vi "Tracking_voltmeter.vi"() -> ()   [LabVIEW 2021]
uses:
  Main states enum-tracking.ctl
  Globals/Global message.vi
  Globals/CH1.vi
  Globals/CH2.vi
  Globals/CH3.vi
  Globals/CH4.vi
  Globals/CH5.vi
panel:
  in  "Time base [ms]":u32=100
  out "DOWN":bool
  out "UP":bool
  in  "ADC resolution":i32=5
  in  "ADC ref":dbl=5.0
  in  "Input channel":enum16{"CH1", "CH2", "CH3", "CH4", "CH5"}(ring)
  out "Waveform Chart":dynamicdata(graph)=[{"t0"=timestamp(3758015842.540576 s since 1904-01-01), "dt"=1.0, "Y"=[1.9925690374558243]}, {"t0"=timestamp(3758015842.540576 s since 1904-01-01), "dt"=1.0, "Y"=[2.03125]}]
  out "Uo ADC":dbl format="%_3g"
  out "Brojac":i32
  out "Indicator":dbl format="%_3g"
  in  "Stop Button":bool
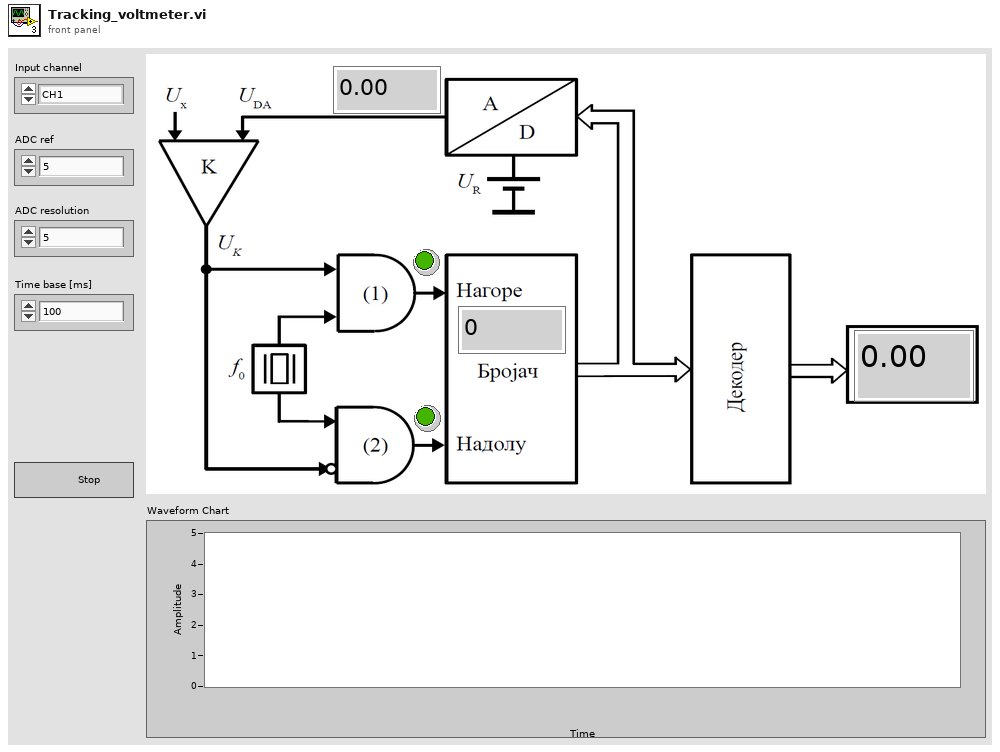
[diagram p1: front panel]
types:
  T1 = typedef "Main states enum-tracking.ctl" = enum16{"Initialize", "Update", "Stop"}
  T2 = cluster{"Voltage":dbl, "Current":dbl, "Message":string}
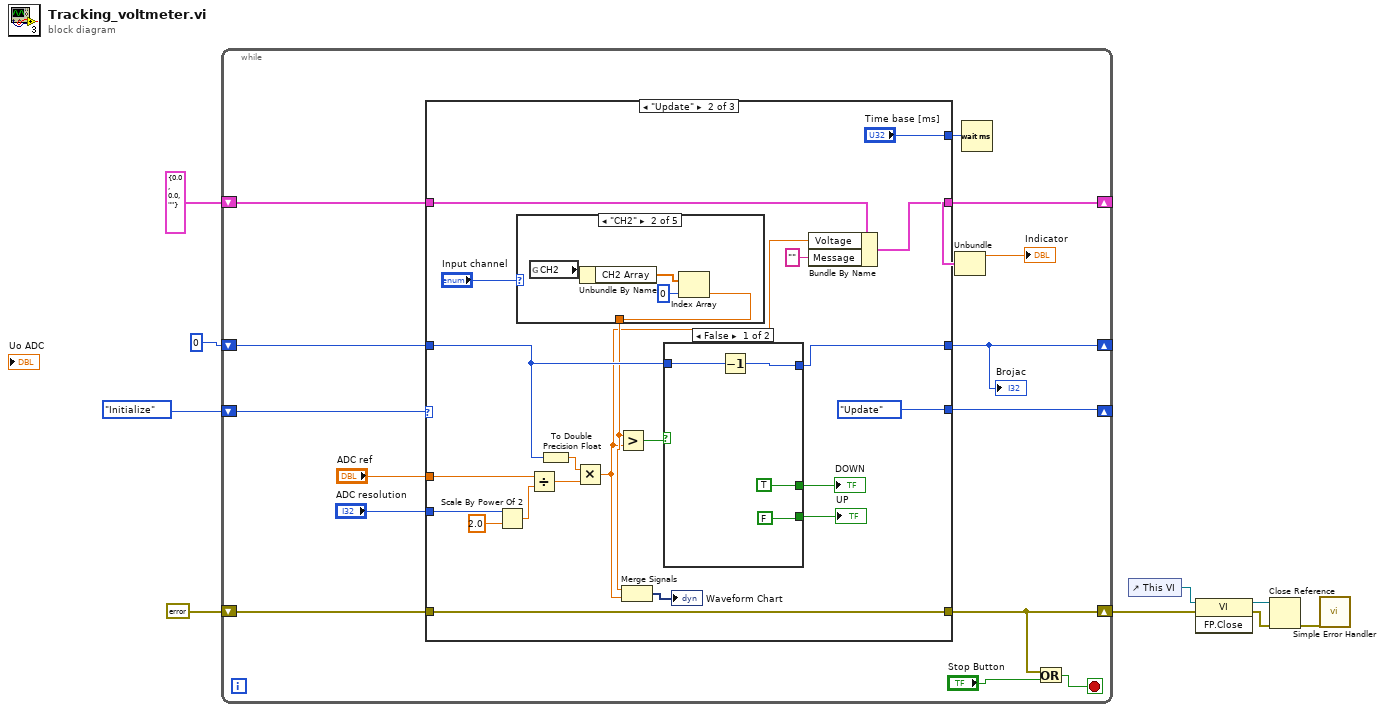
[diagram p0: block diagram]
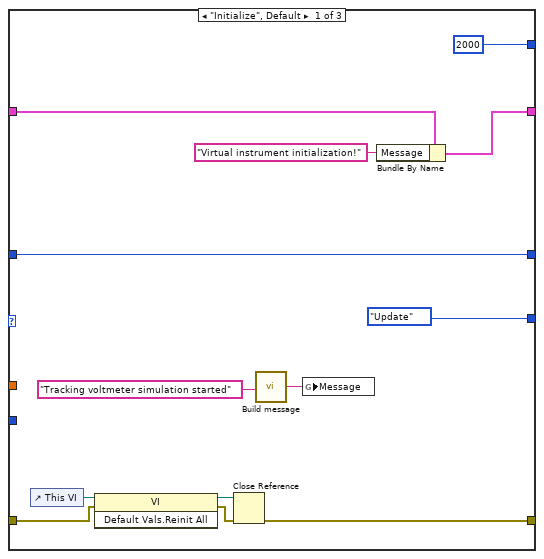
[diagram p2: hidden frame]
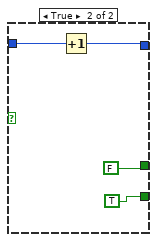
[diagram p3: hidden frame]
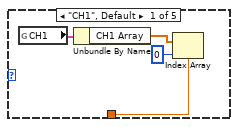
[diagram p4: hidden frame]
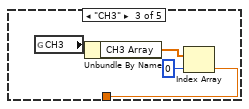
[diagram p5: hidden frame]
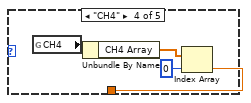
[diagram p6: hidden frame]
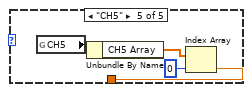
[diagram p7: hidden frame]
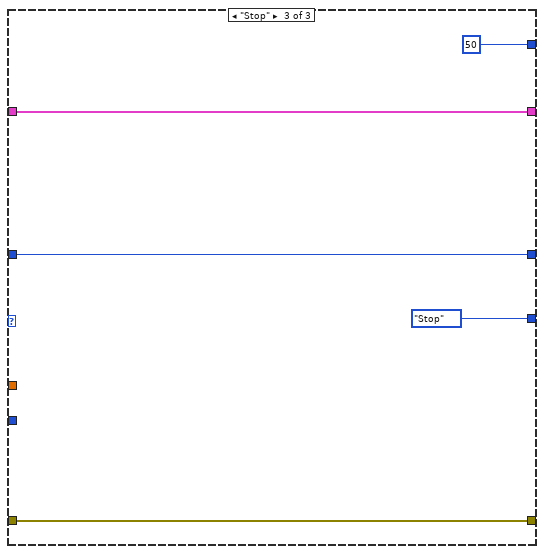
[diagram p8: hidden frame]
diagram:
  n1 = while {
    shift-right: [w21] -> w8
    shift-left: errorcluster {"status"=FALSE, "code"=0, "source"=""} ("error constant") -> [w23]
    shift-right: [w17] -> _
    shift-left: T2 {"Voltage"=0.0, "Current"=0.0, "Message"=""} -> [w20]
    shift-right: [w18] -> _
    shift-left: Main_states_enum-tracking."Initialize" ("Enum") -> [w19]
    shift-right: [w10] -> _
    shift-left: 0 -> [w11]
    stop <- w22 stop-if-true
    n2 = case shown="\"Update\"" w19 {
      tunnel: w23 -> [w33 w57 w90]
      tunnel: [w28 w57 w90] -> w21
      tunnel: w20 -> [w30 w54 w88]
      tunnel: [w29 w56 w88] -> w17
      tunnel: [Main_states_enum-tracking."Update" ("Enum") Main_states_enum-tracking."Update" ("Enum") Main_states_enum-tracking."Stop" ("Enum")] -> w18
      tunnel: [u32 2000 ("milliseconds to wait") "Time base [ms]" u32 50 ("milliseconds to wait")] -> w16
      tunnel: "ADC ref" -> [_ w50 _]
      tunnel: "ADC resolution" -> [_ w49 _]
      tunnel: w11 -> [w24 w43 w86]
      tunnel: [w24 w42 w86] -> w10
      frame "Initialize", Default {
        n3 = control-ref of="This VI"() -> (w36:refnum<vi>)
        n4 = invoke class="VI" method="Default Vals.Reinit All"(reference=w36, error in=w33) -> (reference out=w35:refnum<vi>, error out=w34:errorcluster)  [unwired: 1 in, 1 out]
        n5 = Close Reference(reference=w35, error in (no error)=w34) -> (error out=w28:errorcluster)
        n6 = call "Build message.vi"("Input string"="Tracking voltmeter simulation started") -> ("Output string"=w26:string)
        n7 = global write "Global message.vi" "Message"(w26) -> ()
        n8 = Bundle By Name(cluster=w30, "Message"="Virtual instrument initialization!") -> (w29:T2)
      }
      frame "Update" {
        n9 = Scale By Power Of 2(n=w49, x=2.0) -> (x*2^n=w47:dbl)
        n10 = case shown="\"CH2\"" "Input channel" {
          tunnel: [w66 w70 w74 w78 w82] -> w40
          frame "CH1", Default {
            n11 = global read "CH1.vi" "CH1"() -> (w69:cluster{"CH1 Array":dbl[], "CH1 Message":string})
            n12 = Unbundle By Name(w69) -> ("CH1 Array"=w68:dbl[])
            n13 = Index Array(array=w68, index=0) -> (element=w66:dbl)
          }
          frame "CH2" {
            n14 = global read "CH2.vi" "CH2"() -> (w71:cluster{"CH2 Array":dbl[], "CH2 Message":string})
            n15 = Unbundle By Name(w71) -> ("CH2 Array"=w73:dbl[])
            n16 = Index Array(array=w73, index=0) -> (element=w70:dbl)
          }
          frame "CH3" {
            n17 = global read "CH3.vi" "CH3"() -> (w75:cluster{"CH3 Array":dbl[], "CH3 Message":string})
            n18 = Unbundle By Name(w75) -> ("CH3 Array"=w77:dbl[])
            n19 = Index Array(array=w77, index=0) -> (element=w74:dbl)
          }
          frame "CH4" {
            n20 = global read "CH4.vi" "CH4"() -> (w79:cluster{"CH4 Array":dbl[], "CH4 Message":string})
            n21 = Unbundle By Name(w79) -> ("CH4 Array"=w81:dbl[])
            n22 = Index Array(array=w81, index=0) -> (element=w78:dbl)
          }
          frame "CH5" {
            n23 = global read "CH5.vi" "CH5"() -> (w83:cluster{"CH5 Array":dbl[], "CH5 Message":string})
            n24 = Unbundle By Name(w83) -> ("CH5 Array"=w85:dbl[])
            n25 = Index Array(array=w85, index=0) -> (element=w82:dbl)
          }
        }
        n26 = Divide(x=w50, y=w47) -> (x/y=w46:dbl)
        n27 = To Double Precision Float(number=w43) -> (double precision float=w45:dbl)
        n28 = Multiply(x=w45, y=w46) -> (x*y=w39:dbl)
        n29 = Greater?(x=w40, y=w39) -> (0:w44:bool)
        n30 = Merge Signals(w40, w39) -> (→"Waveform Chart":dynamicdata)
        n31 = case shown="False" w44 {
          tunnel: w43 -> [w61 w65]
          tunnel: [w60 w64] -> w42
          tunnel: [TRUE FALSE] -> w38
          tunnel: [FALSE TRUE] -> w37
          frame False {
            n32 = Decrement(x=w61) -> (x-1=w60:i32)
          }
          frame True {
            n33 = Increment(x=w65) -> (x+1=w64:i32)
          }
        }
        "DOWN" <- w38
        "UP" <- w37
        n34 = Bundle By Name(cluster=w54, "Voltage"=w39, "Message"="") -> (w56:T2)
      }
      frame "Stop" {
      }
    }
    "Brojac" <- w10
    n35 = Unbundle(w17) -> ("Voltage"=→"Indicator":dbl)  [unwired: 2 out]
    n36 = Wait (ms)(milliseconds to wait=w16) -> ()  [unwired: 1 out]
    n37 = Or(x=w21, y="Stop Button") -> (x .or. y?=w22:bool)
  }
  n38 = control-ref of="This VI"() -> (w5:refnum<vi>)
  n39 = invoke class="VI" method="FP.Close"(reference=w5, error in=w8) -> (reference out=w3:refnum<vi>, error out=w4:errorcluster)  [unwired: 1 in, 1 out]
  n40 = Close Reference(reference=w3, error in (no error)=w4) -> (error out=w7:errorcluster)
  n41 = call <vilib>:"Simple Error Handler.vi"("error in (no error)"=w7) -> ()  [unwired: 4 in, 5 out]
